vi "UserInterface.vi"() -> ()   [LabVIEW 2012]
uses:
  <vilib>/Rock Robotics/WPI/Joystick/WPI_JoystickGetSetRefNum.vi
  <vilib>/Rock Robotics/WPI/RobotDrive/WPI_RobotDriveOpen4MotorWithExistingMotors.vi
  <vilib>/Rock Robotics/WPI/RobotDrive/WPI_RobotDriveMecanumDrive_Cartesian.vi
panel:
  in  "ShooterDeadBand":dbl=-0.1
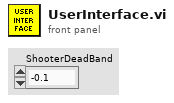
[diagram p1: front panel]
types:
  T1 = typedef "WPI_JoystickDevRef.ctl" = cluster{"Device":T2}
  T2 = typedef "WPI_JoystickDeviceEnum.ctl" = enum16{"USB 1", "USB 2", "USB 3", "USB 4", "Kinect 1", "Kinect 2"}
  T3 = cluster{"axis 1 (x)":dbl, "axis 2 (y)":dbl, "axis 3 (throttle)":dbl, "axis 4":dbl, "axis 5":dbl, "axis 6":dbl}
  T4 = typedef "WPI_MotorControlDeviceRef.ctl" = cluster{"DeviceStatus":errorcluster, "Type":enum16{"PWM", "CAN"}, "PWM":cluster{"Digital Module":T5, "PWM Channel":T6, "DeadBand":T7}, "CAN":cluster{"Device Number":u8, "Control Mode":T8, "Semaphore":T9, "Max Vout":dbl}, "Invert":bool, "TransformRef":T10, "InvTransformRef":T10}
  T5 = typedef "FPGA_TypedefDigitalModule.ctl" = enum16{"Digital Module 1", "Digital Module 2"}
  T6 = typedef "FPGA_DIOPWMChannel.ctl" = enum8{"PWM 1", "PWM 2", "PWM 3", "PWM 4", "PWM 5", "PWM 6", "PWM 7", "PWM 8", "PWM 9", "PWM 10", "Invalid"}
  T7 = typedef "WPI_PWMDeadband.ctl" = cluster{"Name":string, "maxPositivePwm":i32, "minPositivePwm":i32, "centerPwm":i32, "maxNegativePwm":i32, "minNegativePwm":i32, "angularRange":u16}
  T8 = typedef "WPI_CANJaguar_ControlMode.ctl" = enum8{"Percent VBus", "Current", "Speed", "Position", "Voltage"}
  T9 = typedef "Semaphore RefNum" = refnum<k1>
  T10 = typedef "WPI_PWMTransform_ConPane.ctl" = refnum<vi>
  T11 = typedef "WPI_RobotDriveDevRef.ctl" = cluster{"DevStatus":errorcluster, "Motors[]":T4[], "Square Inputs":bool, "Max Output":dbl, "Isochronous":bool}
  T12 = typedef "WPI_JoystickButtonState.ctl" = cluster{"Button 1":bool, "Button 2":bool, "Button 3":bool, "Button 4":bool, "Button 5":bool, "Button 6":bool, "Button 7":bool, "Button 8":bool, "Button 9":bool, "Button 10":bool, "Button 11":bool, "Button 12":bool}
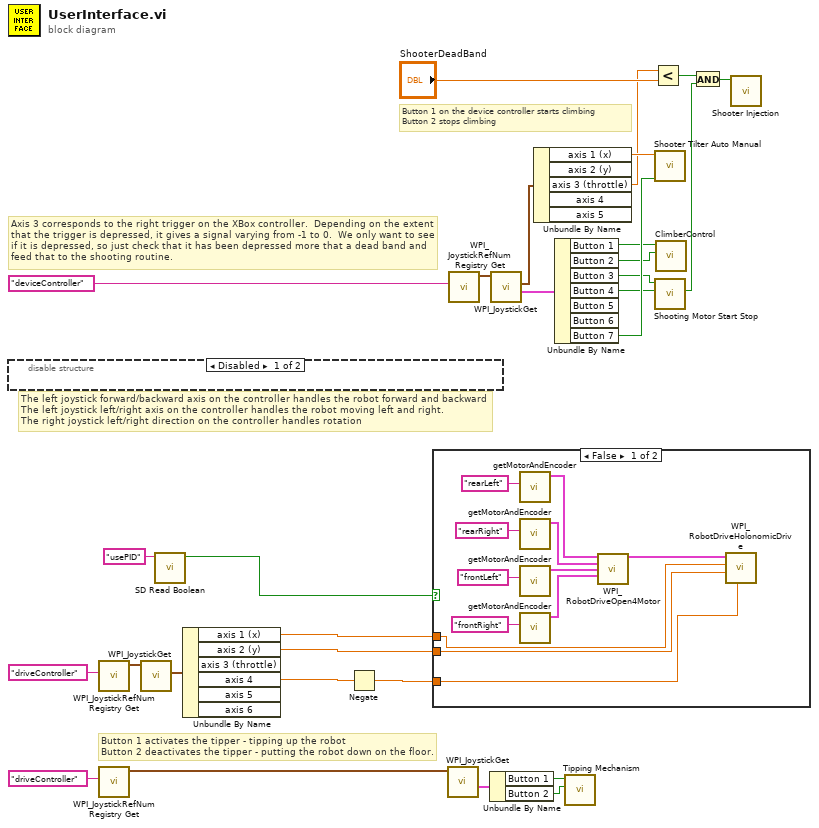
[diagram p0: block diagram]
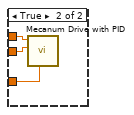
[diagram p2: hidden frame]
diagram:
  # "The left joystick forward/backward axis on the controller handles the robot forward and backward\nThe left joystick left/right axis on the controller handles the robot moving left and right.\nThe right joystick left/right direction on the controller handles rotation"
  # "Button 1 activates the tipper - tipping up the robot\nButton 2 deactivates the tipper - putting the robot down on the floor."
  # "Button 1 on the device controller starts climbing\nButton 2 stops climbing"
  # "Axis 3 corresponds to the right trigger on the XBox controller.  Depending on the extent\nthat the trigger is depressed, it gives a signal varying from -1 to 0.  We only want to see\nif it is depressed, so just check that it has been depressed more that a dead band and \nfeed that to the shooting routine."
  n1 = disable-structure shown="Disabled" {
    frame Disabled {
    }
    frame Enabled {
    }
  }
  n2 = call <vilib>:"WPI_JoystickRefNum Registry Get.vi"("refnum name"="driveController") -> ("JoystickDevRef"=w16:T1)  [unwired: 1 in, 9 out]
  n3 = call <vilib>:"WPI_JoystickRefNum Registry Get.vi"("refnum name"="driveController") -> ("JoystickDevRef"=w21:T1)  [unwired: 9 in, 1 out]
  n4 = call <vilib>:"WPI_JoystickGet.vi"("JoystickDevRef"=w16) -> ("Axes"=w15:T3)  [unwired: 1 in, 5 out]
  n5 = call <vilib>:"SD Read Boolean.vi"("Name"="usePID") -> ("Boolean"=w6:bool)  [unwired: 8 in, 2 out]
  n6 = Unbundle By Name(w15) -> ("axis 1 (x)"=w8:dbl, "axis 2 (y)"=w7:dbl, "axis 4"=w4:dbl)  [unwired: 3 out]
  n7 = Negate(x=w4) -> (-x=w3:dbl)
  n8 = case shown="False" w6 {
    tunnel: w3 -> [w30 w44]
    tunnel: w8 -> [w32 w43]
    tunnel: w7 -> [w31 w42]
    frame False {
      n9 = call "getMotorAndEncoder.vi"("Name"="rearLeft") -> ("MotorControlDevRef"=w36:T4)  [unwired: 8 in, 2 out]
      n10 = call "getMotorAndEncoder.vi"("Name"="rearRight") -> ("MotorControlDevRef"=w37:T4)  [unwired: 8 in, 2 out]
      n11 = call "getMotorAndEncoder.vi"("Name"="frontLeft") -> ("MotorControlDevRef"=w35:T4)  [unwired: 8 in, 2 out]
      n12 = call "getMotorAndEncoder.vi"("Name"="frontRight") -> ("MotorControlDevRef"=w34:T4)  [unwired: 8 in, 2 out]
      n13 = call-poly <vilib>:"WPI_RobotDriveOpen4Motor.vi"("Rear Left Motor Dev Ref"=w36, "Rear Right Motor Dev Ref"=w37, "Front Left Motor Dev Ref"=w35, "Front Right Motor Dev Ref"=w34) -> ("RobotDriveDevRef"=w33:T11)  [unwired: 10 in, 1 out]
      n14 = call-poly <vilib>:"WPI_RobotDriveHolonomicDrive.vi"("Rotation"=w30, "Y"=w31, "X"=w32, "RobotDriveDevRef"=w33) -> ()  [unwired: 5 in, 3 out]
    }
    frame True {
      n15 = call "Mecanum Drive with PID.vi"("Rotation"=w44, "Y"=w42, "X"=w43) -> ()  [unwired: 9 in]
    }
  }
  n16 = call <vilib>:"WPI_JoystickGet.vi"("JoystickDevRef"=w21) -> ("Buttons"=w20:T12)  [unwired: 4 in, 2 out]
  n17 = call <vilib>:"WPI_JoystickRefNum Registry Get.vi"("refnum name"="deviceController") -> ("JoystickDevRef"=w28:T1)  [unwired: 9 in, 1 out]
  n18 = Unbundle By Name(w20) -> ("Button 1"=w19:bool, "Button 2"=w18:bool)
  n19 = call <vilib>:"WPI_JoystickGet.vi"("JoystickDevRef"=w28) -> ("Buttons"=w27:T12, "Axes"=w26:T3)  [unwired: 4 in, 1 out]
  n20 = Unbundle By Name(w26) -> ("axis 1 (x)"=w24:dbl, "axis 3 (throttle)"=w14:dbl)  [unwired: 3 out]
  n21 = Unbundle By Name(w27) -> ("Button 1"=w1:bool, "Button 2"=w2:bool, "Button 3"=w13:bool, "Button 4"=w12:bool, "Button 7"=w23:bool)  [unwired: 2 out]
  n22 = call "Tipping Mechanism.vi"("Un-Tip"=w18, "Tip"=w19) -> ()  [unwired: 10 in]
  n23 = Less?(x=w14, y="ShooterDeadBand") -> (x < y?=w10:bool)
  n24 = call "Shooter Tilter Auto Manual.vi"("changeMode"=w23, "joystickNumber"=w24) -> ()  [unwired: 10 in]
  n25 = call "Shooting Motor Start Stop.vi"("Stop"=w12, "Start"=w13) -> ("Ready To Shoot"=w11:bool)  [unwired: 9 in]
  n26 = call "ClimberControl.vi"("Down"=w2, "Up"=w1) -> ()  [unwired: 10 in]
  n27 = And(x=w10, y=w11) -> (x .and. y?=w9:bool)
  n28 = call "Shooter Injection.vi"("Inject"=w9) -> ()  [unwired: 11 in]
